vi "Configure Output.vi"(6 "Output Impedance (0: Open)":u16(ring) items=["Open", "50 Ohms", "600 Ohms"], 7 "Output Filter (0: Auto)":u16(ring) items=["Auto", "Elliptical 10MHz", "Elliptical 16MHz", "Bessel", "None"], 8 "error in (no error)":errorcluster, 9 "Output Operation (1: Normal)":u16(ring)=1 items=["Inverted", "Normal"], 10 "Output Mode (0: Continuous)":u16(ring) items=["Continuous", "Triggered", "Gated", "Sweep", "Tone"], 11 "VISA resource name":refnum<visa-resource-name>) -> (0 "error out":errorcluster, 3 "VISA resource name out":refnum<visa-resource-name>)   [LabVIEW 2015, in "Fluke 28x Series.lvlib"]
doc: "Configures waveform output settings."
uses:
  <instrlib>/Fluke 28x Series/Fluke 28x Series.lvlib
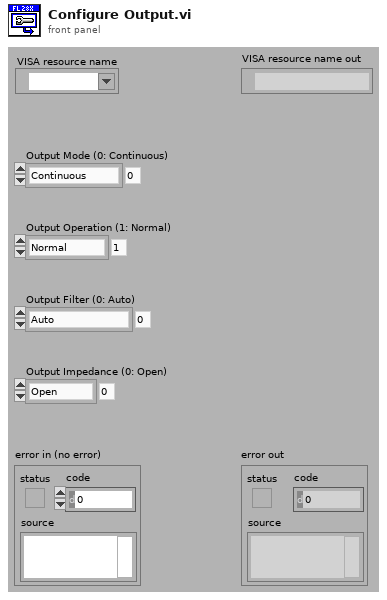
[diagram p1: front panel]
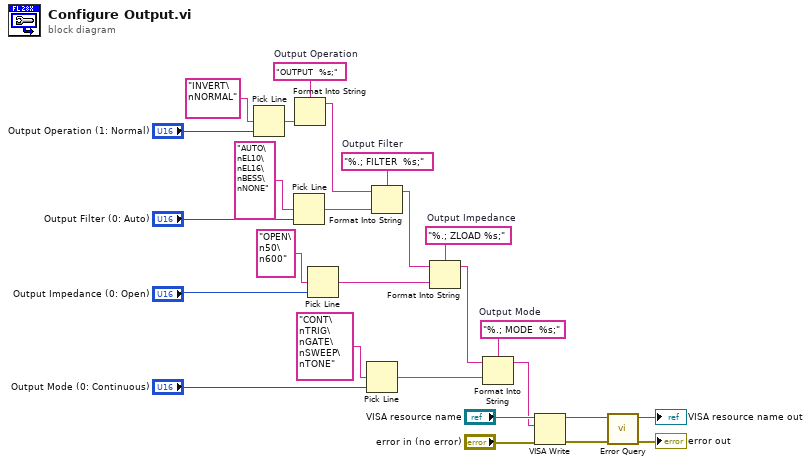
[diagram p0: block diagram]
diagram:
  w3 = "%.; ZLOAD %s;"  # Output Impedance
  w12 = "%.; MODE  %s;"  # Output Mode
  w20 = "%.; FILTER  %s;"  # Output Filter
  w26 = "OUTPUT  %s;"  # Output Operation
  n1 = Pick Line(multi-line string="INVERT\nNORMAL", line index="Output Operation (1: Normal)") -> (output string=w23:string)  [unwired: 1 in]
  n2 = Pick Line(multi-line string="AUTO\nEL10\nEL16\nBESS\nNONE", line index="Output Filter (0: Auto)") -> (output string=w9:string)  [unwired: 1 in]
  n3 = Format Into String(format string=w26, w23) -> (resulting string=w19:string)  [unwired: 2 in, 1 out]
  n4 = Pick Line(multi-line string="OPEN\n50\n600", line index="Output Impedance (0: Open)") -> (output string=w5:string)  [unwired: 1 in]
  n5 = Pick Line(multi-line string="CONT\nTRIG\nGATE\nSWEEP\nTONE", line index="Output Mode (0: Continuous)") -> (output string=w11:string)  [unwired: 1 in]
  n6 = Format Into String(format string=w20, initial string=w19, w9) -> (resulting string=w7:string)  [unwired: 1 in, 1 out]
  n7 = Format Into String(format string=w3, initial string=w7, w5) -> (resulting string=w8:string)  [unwired: 1 in, 1 out]
  n8 = Format Into String(format string=w12, initial string=w8, w11) -> (resulting string=w10:string)  [unwired: 1 in, 1 out]
  n9 = VISA Write(VISA resource name="VISA resource name", write buffer=w10, error in (no error)="error in (no error)") -> (VISA resource name out=w17:refnum<visa-resource-name>, error out=w16:errorcluster)  [unwired: 1 out]
  n10 = call <instrlib>:"Error Query.vi"("error in (no error)"=w16, "VISA resource name"=w17) -> ("error out"=→"error out":errorcluster, "VISA resource name out"=→"VISA resource name out":refnum<visa-resource-name>)  [unwired: 6 in, 2 out]
